vi "GetHardpointActuatorDataField.vi"(10 "Telemetry Data":string, 11 "Cluster in":refnum<vi>) -> (3 "Array":string[](array[string]))   [LabVIEW 2016]
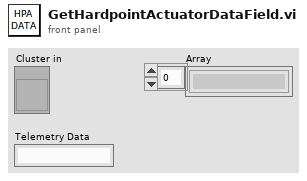
[diagram p1: front panel]
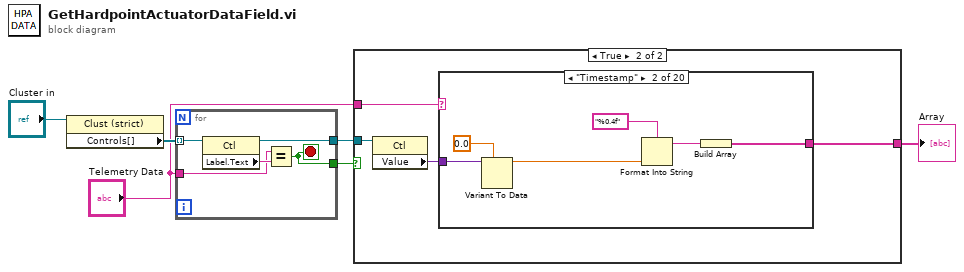
[diagram p0: block diagram]
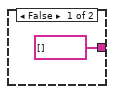
[diagram p2: hidden frame]
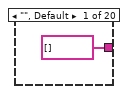
[diagram p3: hidden frame]
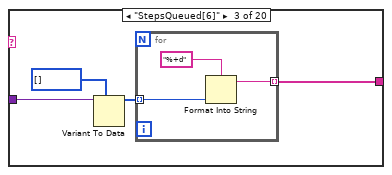
[diagram p4: hidden frame]
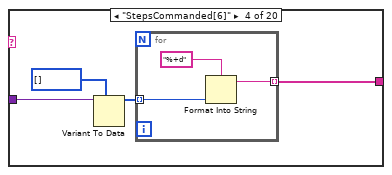
[diagram p5: hidden frame]
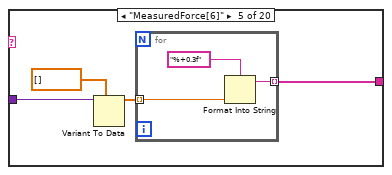
[diagram p6: hidden frame]
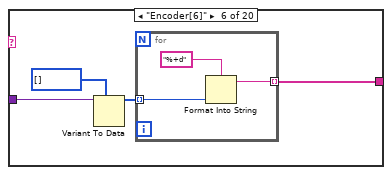
[diagram p7: hidden frame]
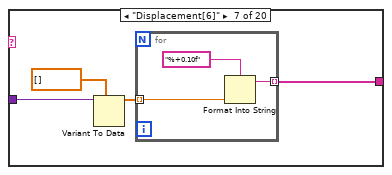
[diagram p8: hidden frame]
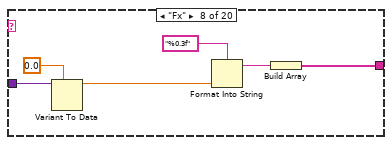
[diagram p9: hidden frame]
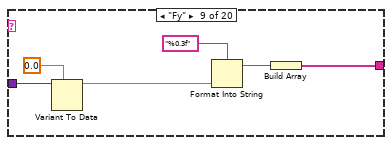
[diagram p10: hidden frame]
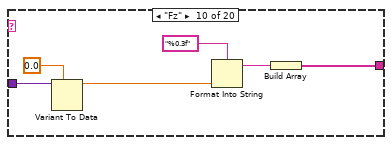
[diagram p11: hidden frame]
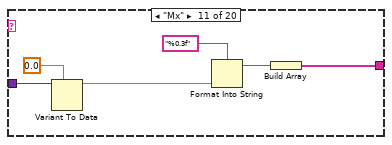
[diagram p12: hidden frame]
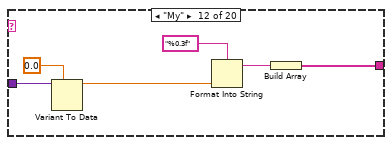
[diagram p13: hidden frame]
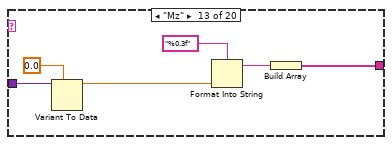
[diagram p14: hidden frame]
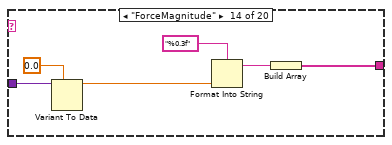
[diagram p15: hidden frame]
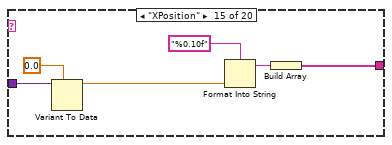
[diagram p16: hidden frame]
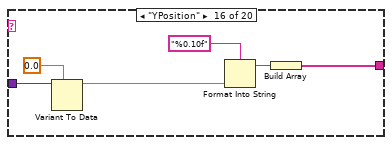
[diagram p17: hidden frame]
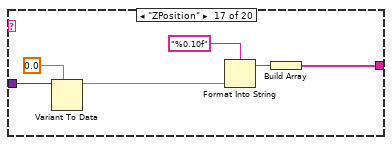
[diagram p18: hidden frame]
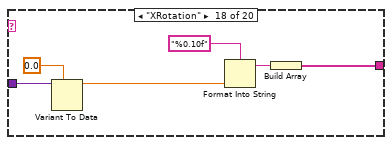
[diagram p19: hidden frame]
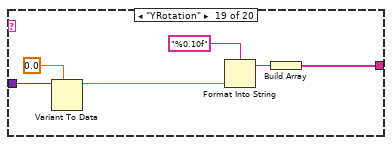
[diagram p20: hidden frame]
diagram:
  n1 = property on="Property Node" class="Clust (strict)"(reference="Cluster in") -> ("Controls[]"=w6:refnum<vi>[])  [unwired: 1 in, 2 out]
  n2 = for {
    tunnel: w6 -> [w11] mode=indexing
    tunnel: [w10] -> w1
    tunnel: "Telemetry Data" -> [w8]
    tunnel: [w7] -> w2
    stop <- w7 stop-if-true
    n3 = property on="Property Node" class="Ctl"(reference=w11) -> (reference out=w10:refnum<vi>, "Label.Text"=w9:string)  [unwired: 1 in, 1 out]
    n4 = Equal?(x=w8, y=w9) -> (x = y?=w7:bool)
  }
  n5 = case shown="True" w2 {
    tunnel: "Telemetry Data" -> [_ w16]
    tunnel: w1 -> [_ w15]
    tunnel: [string[] [] w13] -> w4
    frame False {
    }
    frame True {
      n6 = property on="Property Node" class="Ctl"(reference=w15) -> ("Value"=w14:variant)  [unwired: 1 in, 2 out]
      n7 = case shown="\"Timestamp\"" w16 {
        tunnel: [string[] [] w21 w24 w31 w38 w45 w52 w62 w68 w74 w80 w86 w92 w98 w104 w110 w116 w122 w128 w134] -> w13
        tunnel: w14 -> [_ w19 w27 w34 w41 w48 w55 w60 w66 w72 w78 w84 w90 w96 w102 w108 w114 w120 w126 w132]
        frame "", Default {
        }
        frame "Timestamp" {
          n8 = Variant To Data(type=0.0, Variant=w19) -> (data=w20:dbl)  [unwired: 1 in, 1 out]
          n9 = Format Into String(format string="%0.4f", w20) -> (resulting string=w22:string)  [unwired: 2 in, 1 out]
          n10 = Build Array(w22) -> (w21:string[])
        }
        frame "StepsQueued[6]" {
          n11 = Variant To Data(type=i32[] [], Variant=w27) -> (data=w25:i32[])  [unwired: 1 in, 1 out]
          n12 = for {
            tunnel: w25 -> [w29] mode=indexing
            tunnel: [w28] -> w24 mode=indexing
            n13 = Format Into String(format string="%+d", w29) -> (resulting string=w28:string)  [unwired: 2 in, 1 out]
          }
        }
        frame "StepsCommanded[6]" {
          n14 = Variant To Data(type=i16[] [], Variant=w34) -> (data=w32:i16[])  [unwired: 1 in, 1 out]
          n15 = for {
            tunnel: w32 -> [w36] mode=indexing
            tunnel: [w35] -> w31 mode=indexing
            n16 = Format Into String(format string="%+d", w36) -> (resulting string=w35:string)  [unwired: 2 in, 1 out]
          }
        }
        frame "MeasuredForce[6]" {
          n17 = Variant To Data(type=sgl[] [], Variant=w41) -> (data=w39:sgl[])  [unwired: 1 in, 1 out]
          n18 = for {
            tunnel: w39 -> [w43] mode=indexing
            tunnel: [w42] -> w38 mode=indexing
            n19 = Format Into String(format string="%+0.3f", w43) -> (resulting string=w42:string)  [unwired: 2 in, 1 out]
          }
        }
        frame "Encoder[6]" {
          n20 = Variant To Data(type=i32[] [], Variant=w48) -> (data=w46:i32[])  [unwired: 1 in, 1 out]
          n21 = for {
            tunnel: w46 -> [w50] mode=indexing
            tunnel: [w49] -> w45 mode=indexing
            n22 = Format Into String(format string="%+d", w50) -> (resulting string=w49:string)  [unwired: 2 in, 1 out]
          }
        }
        frame "Displacement[6]" {
          n23 = Variant To Data(type=sgl[] [], Variant=w55) -> (data=w53:sgl[])  [unwired: 1 in, 1 out]
          n24 = for {
            tunnel: w53 -> [w57] mode=indexing
            tunnel: [w56] -> w52 mode=indexing
            n25 = Format Into String(format string="%+0.10f", w57) -> (resulting string=w56:string)  [unwired: 2 in, 1 out]
          }
        }
        frame "Fx" {
          n26 = Variant To Data(type=0.0, Variant=w60) -> (data=w61:dbl)  [unwired: 1 in, 1 out]
          n27 = Format Into String(format string="%0.3f", w61) -> (resulting string=w63:string)  [unwired: 2 in, 1 out]
          n28 = Build Array(w63) -> (w62:string[])
        }
        frame "Fy" {
          n29 = Variant To Data(type=0.0, Variant=w66) -> (data=w67:dbl)  [unwired: 1 in, 1 out]
          n30 = Format Into String(format string="%0.3f", w67) -> (resulting string=w69:string)  [unwired: 2 in, 1 out]
          n31 = Build Array(w69) -> (w68:string[])
        }
        frame "Fz" {
          n32 = Variant To Data(type=0.0, Variant=w72) -> (data=w73:dbl)  [unwired: 1 in, 1 out]
          n33 = Format Into String(format string="%0.3f", w73) -> (resulting string=w75:string)  [unwired: 2 in, 1 out]
          n34 = Build Array(w75) -> (w74:string[])
        }
        frame "Mx" {
          n35 = Variant To Data(type=0.0, Variant=w78) -> (data=w79:dbl)  [unwired: 1 in, 1 out]
          n36 = Format Into String(format string="%0.3f", w79) -> (resulting string=w81:string)  [unwired: 2 in, 1 out]
          n37 = Build Array(w81) -> (w80:string[])
        }
        frame "My" {
          n38 = Variant To Data(type=0.0, Variant=w84) -> (data=w85:dbl)  [unwired: 1 in, 1 out]
          n39 = Format Into String(format string="%0.3f", w85) -> (resulting string=w87:string)  [unwired: 2 in, 1 out]
          n40 = Build Array(w87) -> (w86:string[])
        }
        frame "Mz" {
          n41 = Variant To Data(type=0.0, Variant=w90) -> (data=w91:dbl)  [unwired: 1 in, 1 out]
          n42 = Format Into String(format string="%0.3f", w91) -> (resulting string=w93:string)  [unwired: 2 in, 1 out]
          n43 = Build Array(w93) -> (w92:string[])
        }
        frame "ForceMagnitude" {
          n44 = Variant To Data(type=0.0, Variant=w96) -> (data=w97:dbl)  [unwired: 1 in, 1 out]
          n45 = Format Into String(format string="%0.3f", w97) -> (resulting string=w99:string)  [unwired: 2 in, 1 out]
          n46 = Build Array(w99) -> (w98:string[])
        }
        frame "XPosition" {
          n47 = Variant To Data(type=0.0, Variant=w102) -> (data=w103:dbl)  [unwired: 1 in, 1 out]
          n48 = Format Into String(format string="%0.10f", w103) -> (resulting string=w105:string)  [unwired: 2 in, 1 out]
          n49 = Build Array(w105) -> (w104:string[])
        }
        frame "YPosition" {
          n50 = Variant To Data(type=0.0, Variant=w108) -> (data=w109:dbl)  [unwired: 1 in, 1 out]
          n51 = Format Into String(format string="%0.10f", w109) -> (resulting string=w111:string)  [unwired: 2 in, 1 out]
          n52 = Build Array(w111) -> (w110:string[])
        }
        frame "ZPosition" {
          n53 = Variant To Data(type=0.0, Variant=w114) -> (data=w115:dbl)  [unwired: 1 in, 1 out]
          n54 = Format Into String(format string="%0.10f", w115) -> (resulting string=w117:string)  [unwired: 2 in, 1 out]
          n55 = Build Array(w117) -> (w116:string[])
        }
        frame "XRotation" {
          n56 = Variant To Data(type=0.0, Variant=w120) -> (data=w121:dbl)  [unwired: 1 in, 1 out]
          n57 = Format Into String(format string="%0.10f", w121) -> (resulting string=w123:string)  [unwired: 2 in, 1 out]
          n58 = Build Array(w123) -> (w122:string[])
        }
        frame "YRotation" {
          n59 = Variant To Data(type=0.0, Variant=w126) -> (data=w127:dbl)  [unwired: 1 in, 1 out]
          n60 = Format Into String(format string="%0.10f", w127) -> (resulting string=w129:string)  [unwired: 2 in, 1 out]
          n61 = Build Array(w129) -> (w128:string[])
        }
        frame "ZRotation" {
          n62 = Variant To Data(type=0.0, Variant=w132) -> (data=w133:dbl)  [unwired: 1 in, 1 out]
          n63 = Format Into String(format string="%0.10f", w133) -> (resulting string=w135:string)  [unwired: 2 in, 1 out]
          n64 = Build Array(w135) -> (w134:string[])
        }
      }
    }
  }
  "Array" <- w4
